vi "fill the pulse memory_8 memors.vi"(10 "memory units":T1={"Memory In"="pulse on memory", "Memory In 2"="", "Memory In 3"="", "Memory In 6"="pulse on memory", "Memory In 4"="pulse on memory", "Memory In 5"="", "Memory In 7"="", "Memory In 8"="pulse on memory"}, 11 "FIFO In":refnum<k21>="fifo pulse from host") -> ()   [LabVIEW 2021]
uses:
  <vilib>/rvi/DataTransferAndStorage/Container/Common/niFpgaContainerExecOnDevCompGetState.vi
  <vilib>/rvi/Emulation/niFpgaEmulationIsFPGAContextNoSignature.vi
  <vilib>/rvi/Emulation/niFpgaSctlEmulationGetInTimedLoop.vi
  <vilib>/rvi/errors/niFpgaSetErrorForExecOnDevCompSimple.vi
  <vilib>/rvi/eio/common/nirviEmuReportErrorAndStop.vi
  <vilib>/rvi/DataTransferAndStorage/Container/Common/niFpgaContainerGetUniqueNameForEmu.vi
  <vilib>/rvi/FIFO/Fifo_Resource/nirvififoEmulationSetSize.vi
  <vilib>/rvi/FIFO/Fifo_Resource/nirviFifoEmulationQueueMgr.vi
  <instcachedir>/0/nirviFifoEmulationQueueMgr_E5CAEC123FF24DC58D834DCA3CDAA9B5.lvgen/nirviFifoEmulationQueueMgr_E5CAEC123FF24DC58D834DCA3CDAA9B5_008.vi
  <vilib>/rvi/FIFO/Fifo_Resource/nirvififoEmulationDetermineInputValidOut.vi
  <vilib>/rvi/FIFO/Fifo_Resource/nirvififoEmulationCreateLock.vi
  <vilib>/rvi/Emulation/niFpgaProcessEmulError.vi
  <vilib>/rvi/FIFO/Fifo_Resource/nirvififoEmulationObtainLock.vi
  <vilib>/rvi/FIFO/Fifo_Resource/nirvififoEmulationReleaseLock.vi
  <vilib>/rvi/occurrence/nirviWaitOnOccurrenceBase.vi
  <vilib>/rvi/errors/nirviReportUnexpectedCaseInternalError.vi
  <vilib>/rvi/errors/nirviReportUnexpectedCaseInternalError (U32).vi
  <vilib>/Utility/error.llb/Clear Errors.vi
  <vilib>/rvi/interface/RandomDataEmulation/niFpgaRandomDataHandleErrors.vi
  <vilib>/rvi/Memory/Memory_Emulation/niFpgaMemoryEmulationCacheClearOnFirstRun.vi
  <vilib>/rvi/Memory/Memory_Emulation/nirvimemoryEmulationManagerCache_MakeExclusive.vi
  <vilib>/rvi/Memory/Memory_Emulation/niFpgaMemoryEmulationValidateCache.vi
  <vilib>/rvi/Memory/Memory_Emulation/nirvimemoryEmulationManagerCache_InsertValue.vi
  <vilib>/rvi/Memory/Memory_Emulation/nirvimemoryEmulationManagerCache_ReleaseExclusive.vi
  <vilib>/rvi/Memory/Memory_Emulation/nirvimemoryEmulationManagerCache_GetValue.vi
  <vilib>/rvi/Memory/Memory_Emulation/nirvimemoryEmulationManagerCache_SetValue.vi
  <vilib>/rvi/Emulation/niFpgaSctlEmulationResourceMgr.vi
  <vilib>/rvi/DataTransferAndStorage/Container/XNode/niFpgaContainer.xnode
  <vilib>/rvi/FIFO/Fifo_Resource/niFpgaFifoEmulationRefIn.vi
  <vilib>/rvi/Memory/Memory_Emulation/niFpgaMemoryEmulationRefIn.vi
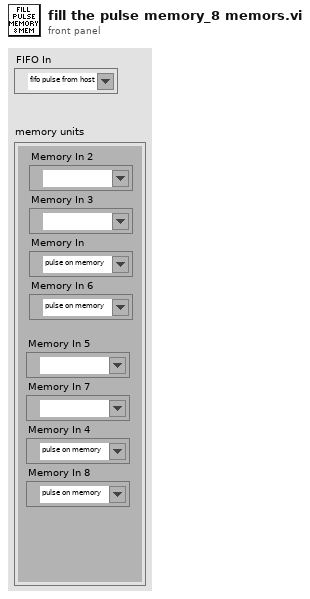
[diagram p1: front panel]
types:
  T1 = cluster{"Memory In":refnum<k21>, "Memory In 2":refnum<k21>, "Memory In 3":refnum<k21>, "Memory In 6":refnum<k21>, "Memory In 4":refnum<k21>, "Memory In 5":refnum<k21>, "Memory In 7":refnum<k21>, "Memory In 8":refnum<k21>}
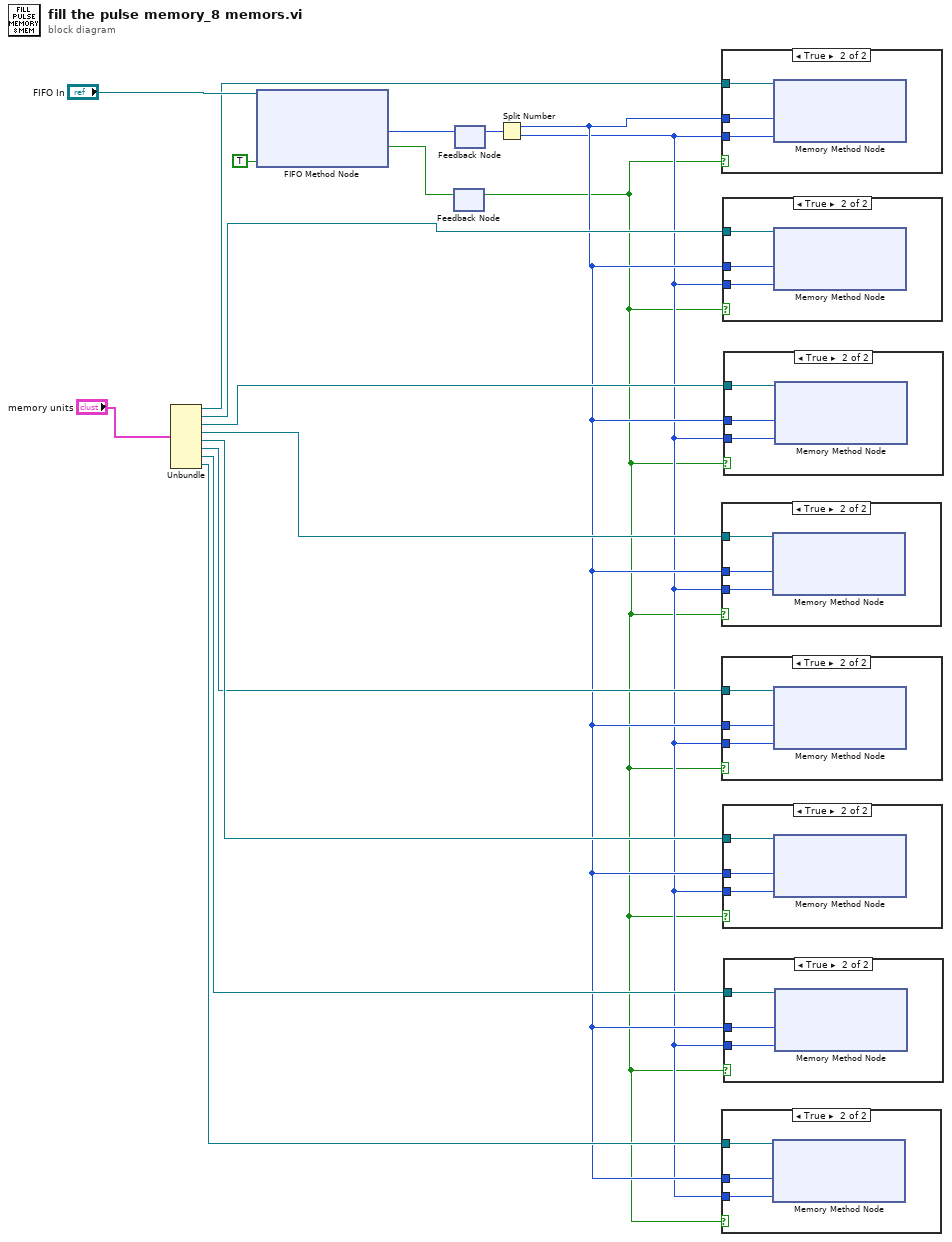
[diagram p0: block diagram]
diagram:
  n1 = Unbundle("memory units") -> ("Memory In"=w14:refnum<k21>, "Memory In 2"=w13:refnum<k21>, "Memory In 3"=w12:refnum<k21>, "Memory In 6"=w11:refnum<k21>, "Memory In 4"=w10:refnum<k21>, "Memory In 5"=w9:refnum<k21>, "Memory In 7"=w8:refnum<k21>, "Memory In 8"=w7:refnum<k21>)
  n2 = xnode ("FIFO Method Node")("Ready for Output"=TRUE, "FIFO In"="FIFO In") -> ("Element"=w2:u64, "Output Valid"=w4:bool)  [unwired: 1 out]
  n3 = feedback-in #1(w4) -> ()
  n4 = feedback #1() -> (w3:bool)  [unwired: 1 in]
  n5 = feedback #2() -> (w1:u64)  [unwired: 1 in]
  n6 = feedback-in #2(w2) -> ()
  n7 = Split Number(x=w1) -> (hi(x)=w6:u32, lo(x)=w5:u32)
  n8 = case shown="True" w3 {
    tunnel: w6 -> [_ w20]
    tunnel: w5 -> [_ w19]
    tunnel: w14 -> [_ w18]
    frame False {
    }
    frame True {
      n9 = xnode ("Memory Method Node")("Address"=w20, "Data"=w19, "Memory In"=w18) -> ()  [unwired: 1 out]
    }
  }
  n10 = case shown="True" w3 {
    tunnel: w6 -> [_ w23]
    tunnel: w5 -> [_ w22]
    tunnel: w11 -> [_ w21]
    frame False {
    }
    frame True {
      n11 = xnode ("Memory Method Node")("Address"=w23, "Data"=w22, "Memory In"=w21) -> ()  [unwired: 1 out]
    }
  }
  n12 = case shown="True" w3 {
    tunnel: w6 -> [_ w26]
    tunnel: w5 -> [_ w25]
    tunnel: w9 -> [_ w24]
    frame False {
    }
    frame True {
      n13 = xnode ("Memory Method Node")("Address"=w26, "Data"=w25, "Memory In"=w24) -> ()  [unwired: 1 out]
    }
  }
  n14 = case shown="True" w3 {
    tunnel: w6 -> [_ w29]
    tunnel: w5 -> [_ w28]
    tunnel: w7 -> [_ w27]
    frame False {
    }
    frame True {
      n15 = xnode ("Memory Method Node")("Address"=w29, "Data"=w28, "Memory In"=w27) -> ()  [unwired: 1 out]
    }
  }
  n16 = case shown="True" w3 {
    tunnel: w6 -> [_ w32]
    tunnel: w5 -> [_ w31]
    tunnel: w13 -> [_ w30]
    frame False {
    }
    frame True {
      n17 = xnode ("Memory Method Node")("Address"=w32, "Data"=w31, "Memory In"=w30) -> ()  [unwired: 1 out]
    }
  }
  n18 = case shown="True" w3 {
    tunnel: w6 -> [_ w35]
    tunnel: w5 -> [_ w34]
    tunnel: w10 -> [_ w33]
    frame False {
    }
    frame True {
      n19 = xnode ("Memory Method Node")("Address"=w35, "Data"=w34, "Memory In"=w33) -> ()  [unwired: 1 out]
    }
  }
  n20 = case shown="True" w3 {
    tunnel: w6 -> [_ w38]
    tunnel: w5 -> [_ w37]
    tunnel: w12 -> [_ w36]
    frame False {
    }
    frame True {
      n21 = xnode ("Memory Method Node")("Address"=w38, "Data"=w37, "Memory In"=w36) -> ()  [unwired: 1 out]
    }
  }
  n22 = case shown="True" w3 {
    tunnel: w6 -> [_ w41]
    tunnel: w5 -> [_ w40]
    tunnel: w8 -> [_ w39]
    frame False {
    }
    frame True {
      n23 = xnode ("Memory Method Node")("Address"=w41, "Data"=w40, "Memory In"=w39) -> ()  [unwired: 1 out]
    }
  }
